vi "Touch and Limit controller Test.vi"(3 "error in (no error)":errorcluster) -> (0 "error out":errorcluster={"status"=TRUE, "code"=1172, "source"="Error calling method Aerotech.A3200.LabVIEW.DiagPacketPoller.Retrieve, (System.Reflection.TargetInvocationException: Exception has been thrown by the target of an invocation.\n\tInner Exception: System.NullReferenceException: Object reference not set to an instance of an object.) <append><b>System.NullReferenceException</b> in RetrieveDiagPacket.vi->Faults and Position data.vi->Aerotech Controller (main).vi"}, 2 "Touching":bool)   [LabVIEW 2016]
uses:
  <vilib>/DAQmx/read.llb/DAQmx Read (Digital Bool 1Line 1Point).vi
  <vilib>/DAQmx/create/channels.llb/DAQmx Create Channel (DI-Digital Input).vi
  <vilib>/DAQmx/miscellaneous.llb/DAQmx Fill In Error Info.vi
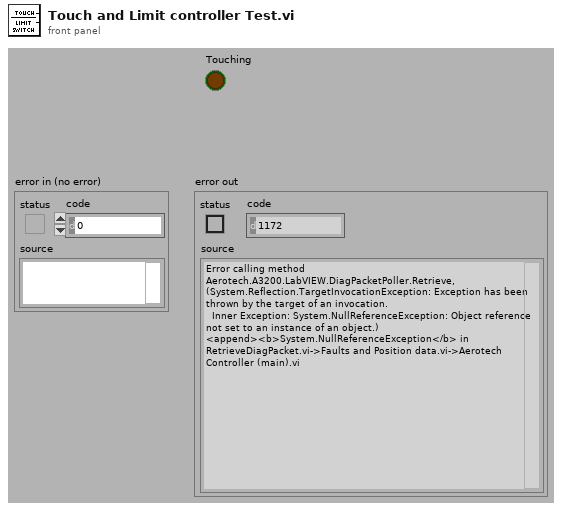
[diagram p1: front panel]
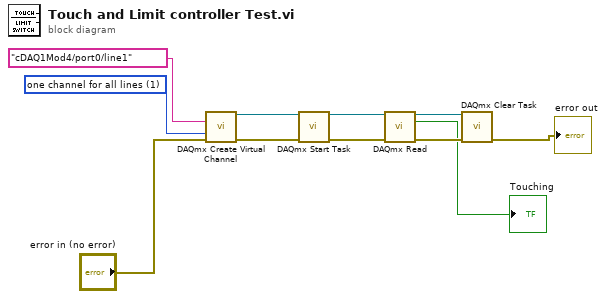
[diagram p0: block diagram]
diagram:
  w10 = 1 items=["one channel for each line", "one channel for all lines"] ("line grouping")
  n1 = call-poly <vilib>:"DAQmx Create Virtual Channel.vi"("lines"=tag "cDAQ1Mod4/port0/line1" ("Lines 2"), "line grouping"=w10, "error in"="error in (no error)") -> ("task out"=w9:refnum<k21>, "error out"=w8:errorcluster)  [unwired: 2 in, 9 out]
  n2 = call <vilib>:"DAQmx Start Task.vi"("task/channels in"=w9, "error in"=w8) -> ("task out"=w7:refnum<k21>, "error out"=w6:errorcluster)  [unwired: 12 out]
  n3 = call-poly <vilib>:"DAQmx Read.vi"("task/channels in"=w7, "error in"=w6) -> ("task out"=w5:refnum<k21>, "data"=→"Touching":bool, "error out"=w4:errorcluster)  [unwired: 11 out]
  n4 = call <vilib>:"DAQmx Clear Task.vi"("task in"=w5, "error in"=w4) -> ("error out"=→"error out":errorcluster)  [unwired: 13 out]
